vi "ZeroStage2.vi"(11 "UiDefinition":T1) -> ()   [LabVIEW 2020]
uses:
  UIReferences.ctl
  C:/Users/User/Desktop/Automation/CurrentVersion/LabviewDXFViewer/bin/Release/LabviewDXFViewer.exe
  LabviewDXFViewer/bin/Release/LabviewDXFViewer.exe
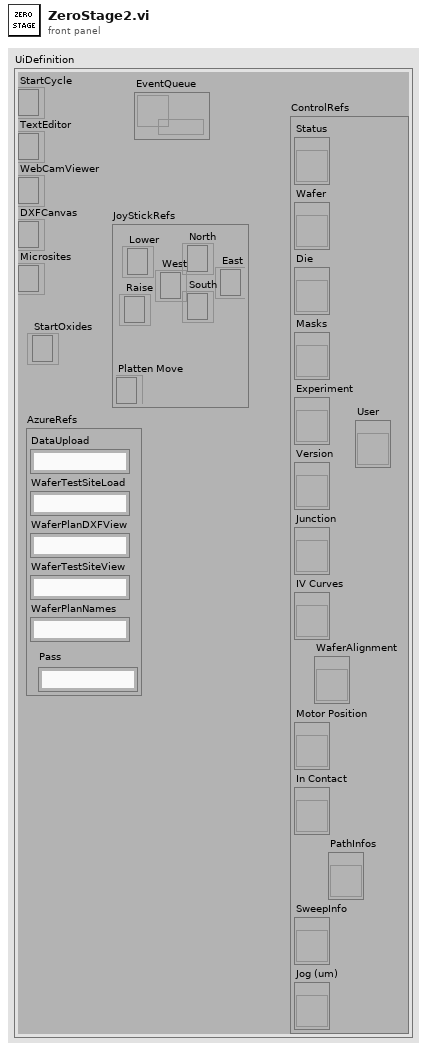
[diagram p1: front panel]
types:
  T1 = typedef "UIReferences.ctl" = cluster{"StartCycle":refnum<k24>, "TextEditor":refnum<k24>, "WebCamViewer":refnum<k24>, "DXFCanvas":refnum<k24>, "Microsites":refnum<k24>, "JoyStickRefs":cluster{"North":refnum<k24>, "Lower":refnum<k24>, "Raise":refnum<k24>, "Platten Move":refnum<k24>, "West":refnum<k24>, "East":refnum<k24>, "South":refnum<k24>}, "AzureRefs":cluster{"DataUpload":string, "WaferTestSiteLoad":string, "WaferPlanDXFView":string, "WaferTestSiteView":string, "WaferPlanNames":string, "Pass":string}, "ControlRefs":cluster{"Status":refnum<vi>, "Wafer":refnum<vi>, "Die":refnum<vi>, "Masks":refnum<vi>, "Experiment":refnum<vi>, "Version":refnum<vi>, "Junction":refnum<vi>, "IV Curves":refnum<vi>, "Motor Position":refnum<vi>, "In Contact":refnum<vi>, "SweepInfo":refnum<vi>, "Jog (um)":refnum<vi>, "PathInfos":refnum<vi>, "User":refnum<vi>, "WaferAlignment":refnum<vi>}, "EventQueue":refnum<queue>, "StartOxides":refnum<k24>}
  T2 = typedef "WaferAlignmentType.ctl" = cluster{"Wafer Units to microns":dbl, "Rotation Misalign":dbl[], "Scale Misalign":dbl, "Steps Per micron":dbl, "Position 1":i32[], "Position 2":i32[], "Lift Distance":i32, "Position 3":i32[], "Jog Height":i32}
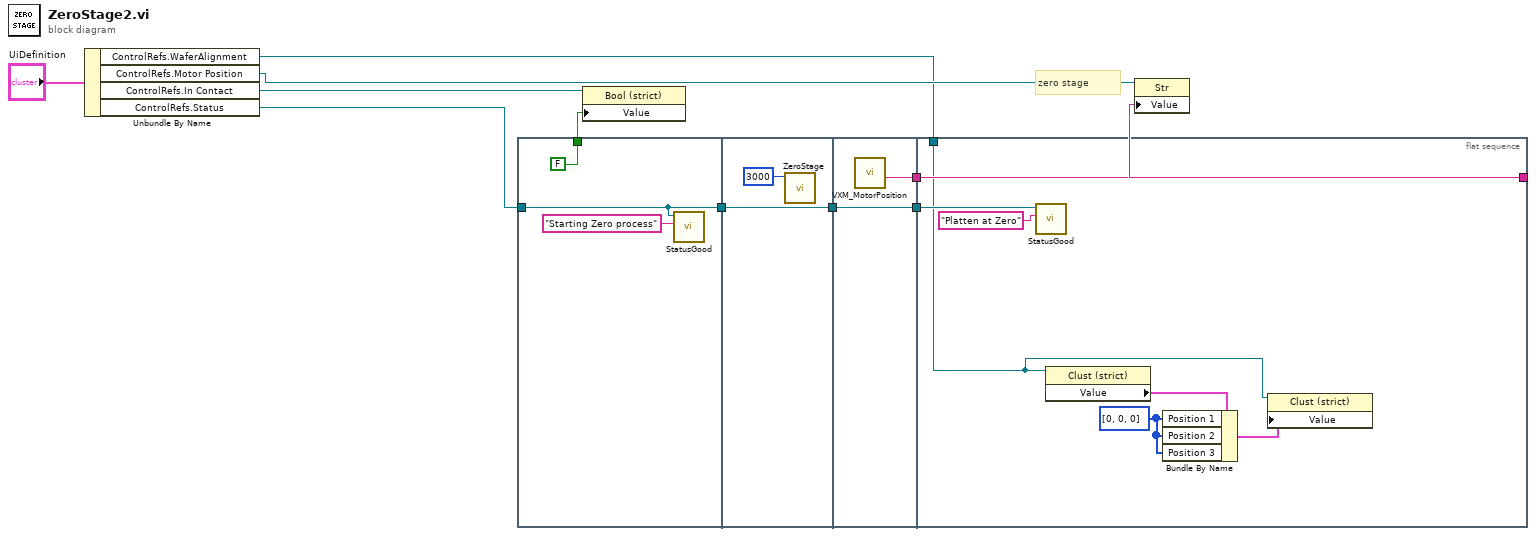
[diagram p0: block diagram]
diagram:
  # "zero stage"
  n1 = Unbundle By Name("UiDefinition") -> ("ControlRefs.WaferAlignment"=w1:refnum<vi>, "ControlRefs.Motor Position"=w5:refnum<vi>, "ControlRefs.In Contact"=w4:refnum<vi>, "ControlRefs.Status"=w2:refnum<vi>)
  n2 = flat-sequence {
    tunnel: w2 -> [w13]
    tunnel: [w13] -> w11
    tunnel: [FALSE ("In Contact")] -> w3
    tunnel: w11 -> [w15]
    tunnel: [w15] -> w10
    tunnel: [w18] -> w9
    tunnel: w10 -> [w17]
    tunnel: [w17] -> w8
    tunnel: [w25] -> w7
    tunnel: w9 -> [w25]
    tunnel: w8 -> [w24]
    tunnel: w1 -> [w19]
    frame #0 {
      n3 = call "StatusGood.vi"("Text.Text"="Starting Zero process", "String in"=w13) -> ()  [unwired: 10 in]
    }
    frame #1 {
      n4 = call "ZeroStage.vi"("milliseconds to wait"=u32 3000) -> ()  [unwired: 11 in]
    }
    frame #2 {
      n5 = call "VXM_MotorPosition.vi"() -> ("Position String"=w18:string)  [unwired: 10 in, 1 out]
    }
    frame #3 {
      w20 = i32[] [0, 0, 0] ("Position 1")
      n6 = call "StatusGood.vi"("Text.Text"="Platten at Zero", "String in"=w24) -> ()  [unwired: 10 in]
      n7 = property class="Clust (strict)"(reference=w19) -> ("Value"=w22:T2)  [unwired: 1 in, 2 out]
      n8 = Bundle By Name(cluster=w22, "Position 1"=w20, "Position 2"=w20, "Position 3"=w20) -> (w21:T2)
      n9 = property class="Clust (strict)"(reference=w19, "Value"=w21) -> ()  [unwired: 1 in, 2 out]
    }
  }
  n10 = property class="Bool (strict)"(reference=w4, "Value"=w3) -> ()  [unwired: 1 in, 2 out]
  n11 = property class="Str"(reference=w5, "Value"=w7) -> ()  [unwired: 1 in, 2 out]
